vi "Init GUI.vi"(11 "Module in":refnum<class "Module.lvclass">) -> (3 "Module out":refnum<class "Module.lvclass">, 5 "Event Reg":refnum<event-registration>)   [LabVIEW 2020, in "Volatus.lvlib" / "Module.lvclass"]
uses:
  Module.lvclass
  GUI Events.ctl
  Module.lvclass/Module.ctl
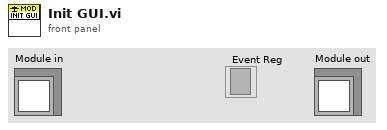
[diagram p1: front panel]
types:
  T1 = typedef "Volatus.lvlib/Module.lvclass/GUI Events.ctl" = cluster{"Close":refnum<user-event>}
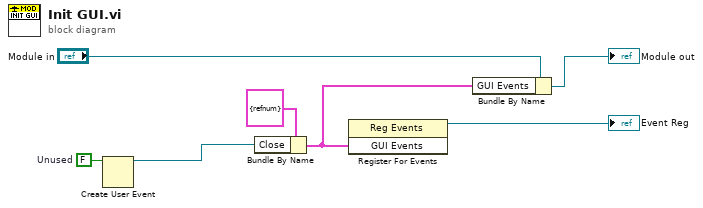
[diagram p0: block diagram]
diagram:
  w5 = FALSE  # Unused
  n1 = Create User Event(user event datatype=w5) -> (user event=w3:refnum<user-event>)  [unwired: 1 in, 1 out]
  n2 = Bundle By Name(cluster=T1 {"Close"=refnum} ("GUI Events"), "Close"=w3) -> (w1:T1)
  n3 = register-events(w1) -> (reference out=→"Event Reg":refnum<event-registration>)  [unwired: 2 in, 1 out]
  n4 = Bundle By Name(cluster="Module in", "GUI Events"=w1) -> (→"Module out":refnum<class "Module.lvclass">)
